vi "Handle Value Change.vi"(5 "VolatusAPI":refnum<class "VolatusAPI.lvclass">, 7 "CtlRef":refnum<vi>, 8 "error in (no error)":errorcluster, 9 "NewVal":variant, 10 "OldVal":variant, 11 "SystemConfigStatusIndicator in":refnum<class "SystemConfigStatusIndicator.lvclass">) -> (0 "error out":errorcluster, 3 "SystemConfigStatusIndicator out":refnum<class "SystemConfigStatusIndicator.lvclass">)   [LabVIEW 2020, in "VolatusGUIElements.lvlib" / "SystemConfigStatusIndicator.lvclass"]
uses:
  SystemConfigStatusIndicator.lvclass
  Volatus/VolatusAPI/VolatusAPI.lvclass
  SystemConfigStatusIndicator.lvclass/SystemConfigStatusIndicator.ctl
  Volatus/Volatus.lvlib
panel:
  out "error out 2":errorcluster
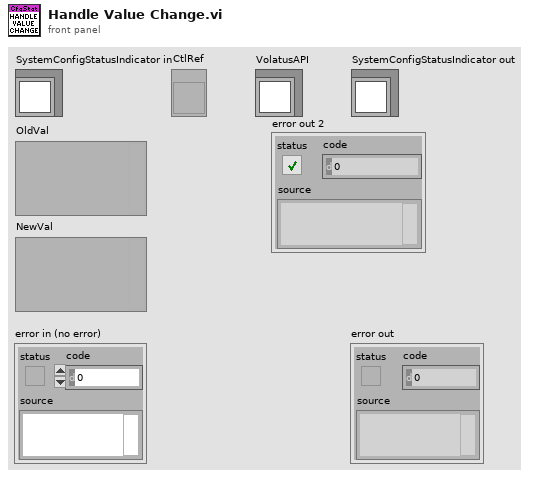
[diagram p1: front panel]
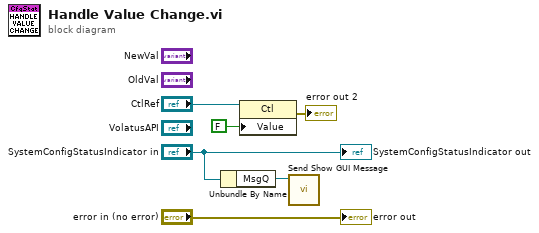
[diagram p0: block diagram]
diagram:
  n1 = Unbundle By Name("SystemConfigStatusIndicator in") -> ("MsgQ"=w2:refnum<class "MessageQ.lvclass">)
  n2 = property class="Ctl"(reference="CtlRef", "Value"=FALSE) -> (error out=→"error out 2":errorcluster)  [unwired: 1 in, 1 out]
  n3 = call "Send Show GUI Message.vi"("MessageQ"=w2) -> ()  [unwired: 10 in, 1 out]
  "error out" <- "error in (no error)"
  "SystemConfigStatusIndicator out" <- "SystemConfigStatusIndicator in"
